vi "Systematic Mutation Change.vi"(8 "error in (no error)":errorcluster, 11 "GA in":refnum<class "GA.lvclass">) -> (0 "error out":errorcluster, 3 "GA out":refnum<class "GA.lvclass">)   [LabVIEW 2013, in "GA.lvclass"]
uses:
  GA.lvclass
  GA.lvclass/GA.ctl
  <vilib>/Analysis/baseanly.llb/Mean (DBL).vi
  <vilib>/Analysis/NI_AALBase.lvlib
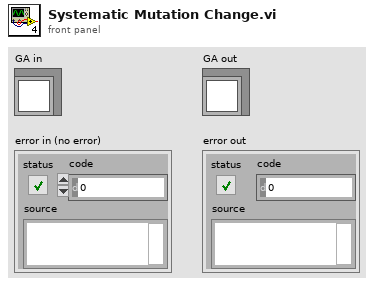
[diagram p1: front panel]
types:
  T1 = typedef "Solution_GA.ctl" = cluster{"Schedule":u16[], "Fitness":u16, "Fitness Valid?":bool}
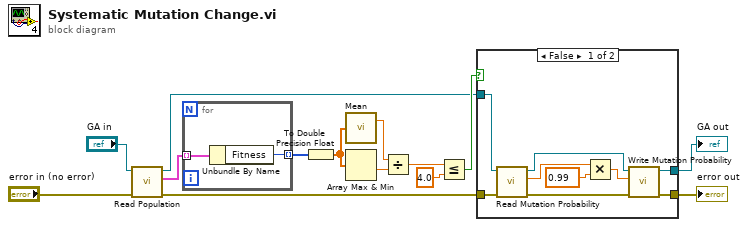
[diagram p0: block diagram]
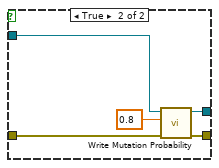
[diagram p2: hidden frame]
diagram:
  n1 = call "Read Population.vi"("error in (no error)"="error in (no error)", "GA in"="GA in") -> ("error out"=w2:errorcluster, "Population"=w10:T1[], "GA out"=w1:refnum<class "GA.lvclass">)  [unwired: 7 in]
  n2 = for {
    tunnel: w10 -> [w16] mode=indexing
    tunnel: [w15] -> w9 mode=indexing
    n3 = Unbundle By Name(w16) -> ("Fitness"=w15:u16)
  }
  n4 = To Double Precision Float(number=w9) -> (double precision float=w8:dbl[])
  n5 = call-poly <vilib>:"Mean.vi"("X"=w8) -> ("mean"=w7:dbl)  [unwired: 1 out]
  n6 = Array Max & Min(array=w8) -> (min value=w6:dbl)  [unwired: 3 out]
  n7 = Divide(x=w7, y=w6) -> (x/y=w5:dbl)
  n8 = Less Or Equal?(x=w5, y=4.0) -> (x <= y?=w3:bool)
  n9 = case shown="False" w3 {
    tunnel: w1 -> [w25 w30]
    tunnel: w2 -> [w22 w29]
    tunnel: [w20 w28] -> w13
    tunnel: [w23 w27] -> w14
    frame False {
      n10 = call "Read Mutation Probability.vi"("error in (no error)"=w22, "GA in"=w25) -> ("error out"=w21:errorcluster, "Mutation Probability"=w19:dbl, "GA out"=w24:refnum<class "GA.lvclass">)  [unwired: 7 in]
      n11 = Multiply(x=w19, y=0.99) -> (x*y=w17:dbl)
      n12 = call "Write Mutation Probability.vi"("error in (no error)"=w21, "Mutation Probability"=w17, "GA in"=w24) -> ("error out"=w20:errorcluster, "GA out"=w23:refnum<class "GA.lvclass">)  [unwired: 7 in]
    }
    frame True {
      n13 = call "Write Mutation Probability.vi"("error in (no error)"=w29, "Mutation Probability"=0.8, "GA in"=w30) -> ("error out"=w28:errorcluster, "GA out"=w27:refnum<class "GA.lvclass">)  [unwired: 7 in]
    }
  }
  "GA out" <- w14
  "error out" <- w13
